vi "Test Bind REP Socket.vi"(8 "error in (no error)":errorcluster, 11 "RemoteControl.ZMQ in":refnum<class "RemoteControl.ZMQ.lvclass">) -> (0 "error out":errorcluster, 3 "RemoteControl.ZMQ out":refnum<class "RemoteControl.ZMQ.lvclass">)   [LabVIEW 2019, in "RemoteControl.ZMQ.lvlib" / "RemoteControl.ZMQ.lvclass"]
uses:
  RemoteControl.ZMQ.lvclass
  <vilib>/addons/_JKI Toolkits/Caraya/classes/Assert/Assert.lvclass
  <vilib>/addons/_JKI Toolkits/Caraya/classes/Assert/Assert Not Error.vi
  <vilib>/addons/zeromq/zmq_context.lvclass
  <vilib>/addons/zeromq/socket_type.ctl
  <vilib>/addons/zeromq/zeromq.lvlib
  <vilib>/addons/zeromq/zmq_socket.lvclass
  <vilib>/addons/_JKI Toolkits/Caraya/classes/Assert/Assert Error.vi
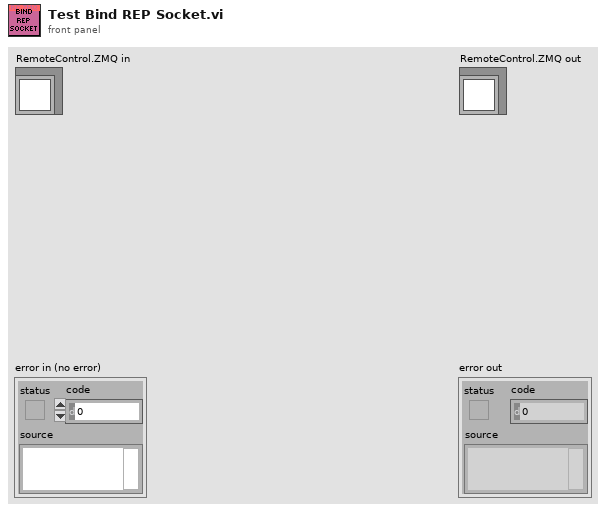
[diagram p1: front panel]
types:
  T1 = typedef "zeromq.lvlib/socket_type.ctl" = enum8{"ZMQ_PAIR", "ZMQ_PUB", "ZMQ_SUB", "ZMQ_REQ", "ZMQ_REP", "ZMQ_DEALER", "ZMQ_ROUTER", "ZMQ_PULL", "ZMQ_PUSH", "ZMQ_XPUB", "ZMQ_XSUB", "ZMQ_STREAM", "ZMQ_SERVER", "ZMQ_CLIENT", "ZMQ_RADIO", "ZMQ_DISH", "ZMQ_GATHER", "ZMQ_SCATTER", "ZMQ_DGRAM"}
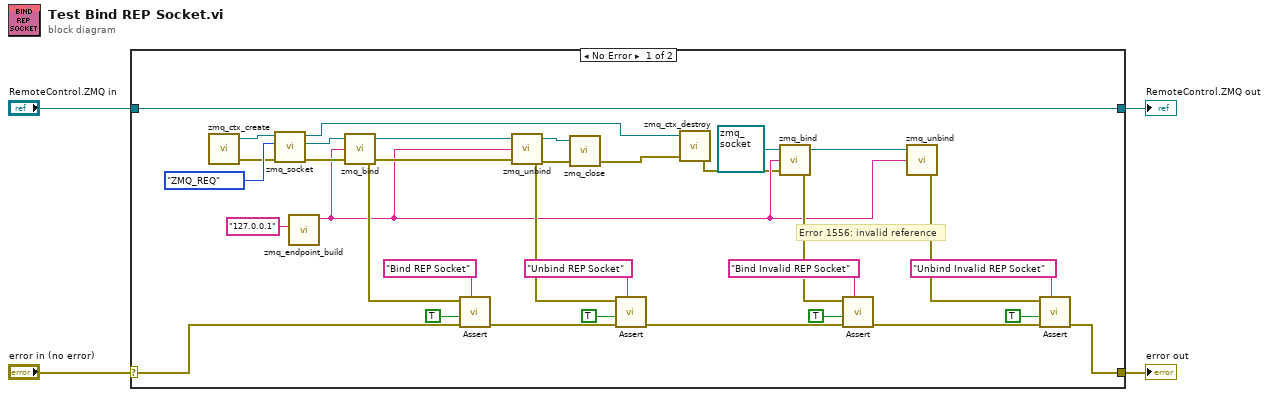
[diagram p0: block diagram]
diagram:
  n1 = case shown="No Error" "error in (no error)" {
    selector: "error in (no error)" -> [w36 w38]
    tunnel: [w7 w38] -> w3
    tunnel: [w33 w37] -> w1
    tunnel: "RemoteControl.ZMQ in" -> [w33 w37]
    frame No Error {
      # "Error 1556: invalid reference"
      n2 = call <vilib>:"zmq_ctx_create.vi"() -> ("error out"=w30:errorcluster, "context out"=w32:refnum<class "zmq_context.lvclass">)  [unwired: 4 in]
      n3 = call <vilib>:"zmq_socket.vi"("error in"=w30, "socket type"=socket_type."ZMQ_REQ", "context in"=w32) -> ("error out"=w29:errorcluster, "socket out"=w28:refnum<class "zmq_socket.lvclass">, "context out"=w20:refnum<class "zmq_context.lvclass">)  [unwired: 2 in]
      n4 = call <vilib>:"zmq_endpoint_build.vi"("address"="127.0.0.1") -> ("endpoint"=w6:string)  [unwired: 4 in, 2 out]
      n5 = call <vilib>:"zmq_bind.vi"("error in"=w29, "endpoint"=w6, "socket in"=w28) -> ("error out"=w26:errorcluster, "socket out"=w27:refnum<class "zmq_socket.lvclass">)  [unwired: 1 in]
      n6 = call-poly <vilib>:"Assert.vi"("Label"="Bind REP Socket", "error in (no error)"=w36, "Register with caller test (F)"=TRUE, "Not Error?"=w26) -> ("error out"=w24:errorcluster)  [unwired: 6 in, 1 out]
      n7 = call <vilib>:"zmq_unbind.vi"("error in"=w26, "endpoint"=w6, "socket in"=w27) -> ("error out"=w21:errorcluster, "socket out"=w23:refnum<class "zmq_socket.lvclass">)  [unwired: 1 in]
      n8 = call <vilib>:"zmq_close.vi"("error in"=w21, "socket"=w23) -> ("error out"=w22:errorcluster)  [unwired: 3 in]
      n9 = call-poly <vilib>:"Assert.vi"("Label"="Unbind REP Socket", "error in (no error)"=w24, "Register with caller test (F)"=TRUE, "Not Error?"=w21) -> ("error out"=w11:errorcluster)  [unwired: 6 in, 1 out]
      n10 = call <vilib>:"zmq_ctx_destroy.vi"("error in"=w22, "context in"=w20) -> ("error out"=w5:errorcluster)  [unwired: 3 in]
      n11 = call <vilib>:"zmq_bind.vi"("error in"=w5, "endpoint"=w6, "socket in"=refnum<class "zmq_socket.lvclass"> refnum) -> ("error out"=w12:errorcluster, "socket out"=w10:refnum<class "zmq_socket.lvclass">)  [unwired: 1 in]
      n12 = call-poly <vilib>:"Assert.vi"("Label"="Bind Invalid REP Socket", "error in (no error)"=w11, "Register with caller test (F)"=TRUE, "Error?"=w12) -> ("error out"=w8:errorcluster)  [unwired: 6 in, 1 out]
      n13 = call <vilib>:"zmq_unbind.vi"("endpoint"=w6, "socket in"=w10) -> ("error out"=w9:errorcluster)  [unwired: 2 in, 1 out]
      n14 = call-poly <vilib>:"Assert.vi"("Label"="Unbind Invalid REP Socket", "error in (no error)"=w8, "Register with caller test (F)"=TRUE, "Error?"=w9) -> ("error out"=w7:errorcluster)  [unwired: 6 in, 1 out]
    }
    frame Error {
    }
  }
  "error out" <- w3
  "RemoteControl.ZMQ out" <- w1
